vi "test_find_elements.vi"() -> ()   [LabVIEW 2018]
uses:
  find_element(array).vi
  find_element(variant).vi
panel:
  out "elapsed time in sec (variant)":dbl
  out "elapsed time in sec (array)":dbl
  in  "number of elements":i32=10000
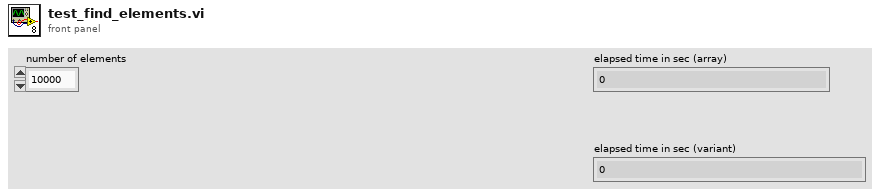
[diagram p1: front panel]
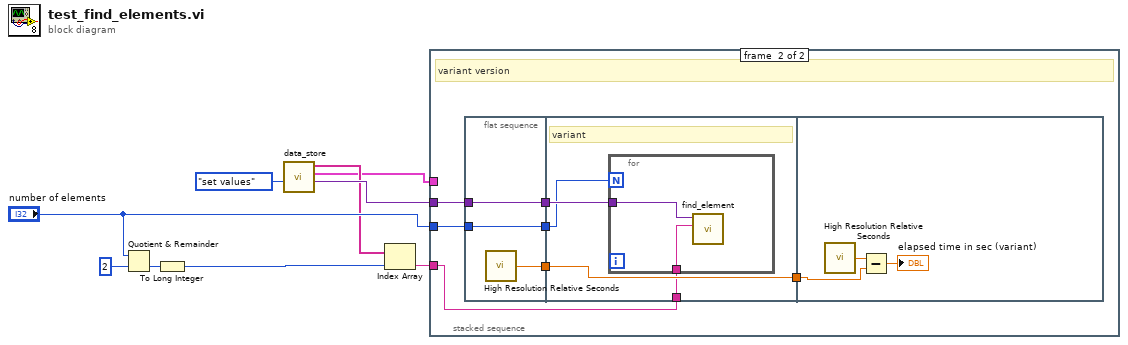
[diagram p0: block diagram]
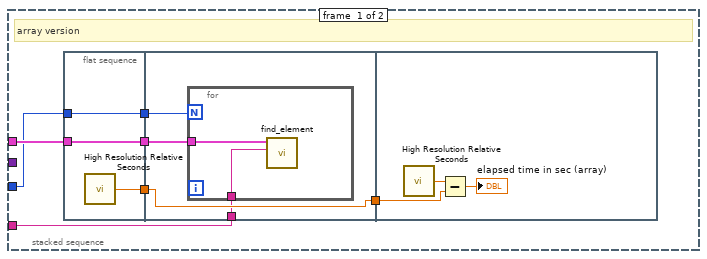
[diagram p2: hidden frame]
diagram:
  n1 = Quotient & Remainder(x="number of elements", y=2) -> (floor(x/y)=w6:i32)  [unwired: 1 out]
  n2 = To Long Integer(number=w6) -> (32bit integer=w3:i32)
  n3 = call "data_store.vi"("Action"=enum16{"set values", "get values"}."set values") -> ("Variant"=w8:variant, "array items"=w1:cluster{"name":string, "address":string}[], "names"=w4:string[])  [unwired: 8 in]
  n4 = Index Array(array=w4, index=w3) -> (element=w2:string)
  n5 = stacked-sequence {
    tunnel: "number of elements" -> [w11 w31]
    tunnel: w1 -> [w13 _]
    tunnel: w8 -> [_ w33]
    tunnel: w2 -> [w12 w29]
    frame #0 {
      # "array version"
      n6 = flat-sequence {
        tunnel: [w19] -> w16
        tunnel: w13 -> [w18]
        tunnel: [w18] -> w15
        tunnel: w11 -> [w17]
        tunnel: [w17] -> w10
        tunnel: [w23] -> w14
        tunnel: w16 -> [w23]
        tunnel: w15 -> [w22]
        tunnel: w12 -> [w21]
        tunnel: w10 -> [w20]
        tunnel: w14 -> [w27]
        frame #0 {
          n7 = call <vilib>:"High Resolution Relative Seconds.vi"() -> ("relative seconds"=w19:dbl)
        }
        frame #1 {
          n8 = for {
            N: w20 -> [_]
            tunnel: w22 -> [w25]
            tunnel: w21 -> [w24]
            n9 = call-poly "find_element.vi"("name"=w24, "data store (in)"=w25) -> ()  [unwired: 6 in, 4 out]
          }
        }
        frame #2 {
          n10 = call <vilib>:"High Resolution Relative Seconds.vi"() -> ("relative seconds"=w28:dbl)
          n11 = Subtract(x=w28, y=w27) -> (x-y=→"elapsed time in sec (array)":dbl)
        }
      }
    }
    frame #1 {
      # "variant version"
      n12 = flat-sequence {
        tunnel: [w38] -> w35
        tunnel: w33 -> [w37]
        tunnel: [w37] -> w32
        tunnel: w31 -> [w36]
        tunnel: [w36] -> w30
        tunnel: [w42] -> w34
        tunnel: w35 -> [w42]
        tunnel: w32 -> [w41]
        tunnel: w30 -> [w40]
        tunnel: w29 -> [w39]
        tunnel: w34 -> [w46]
        frame #0 {
          n13 = call <vilib>:"High Resolution Relative Seconds.vi"() -> ("relative seconds"=w38:dbl)
        }
        frame #1 {
          # "variant"
          n14 = for {
            N: w40 -> [_]
            tunnel: w41 -> [w44]
            tunnel: w39 -> [w43]
            n15 = call-poly "find_element.vi"("name"=w43, "data store (in)"=w44) -> ()  [unwired: 6 in, 4 out]
          }
        }
        frame #2 {
          n16 = call <vilib>:"High Resolution Relative Seconds.vi"() -> ("relative seconds"=w47:dbl)
          n17 = Subtract(x=w47, y=w46) -> (x-y=→"elapsed time in sec (variant)":dbl)
        }
      }
    }
  }
